vi "PH_Beckhoff_StepMot.evt Call Set Axis Configuration.vi"(0 "i ref in":refnum<vi>, 2 "Instance name":string="N/A", 5 "error in":errorcluster) -> (14 "i ref out":refnum<vi>, 19 "error out":errorcluster)   [LabVIEW 2014, in "PH_Beckhoff_StepMot.lvlib"]
doc: "This VI calls an event by a simple call."
uses:
  PH_Beckhoff_StepMot.lvlib
  instr.lib/Beckhoff/Specials/Step Motor Klemmen/Beckhoff.Step Motor - Motor Configuration.ctl
  instr.lib/Beckhoff/Read and Write Register/Step Motor Klemmen/Beckhoff.Step Motor - Feature Register 1.ctl
  instr.lib/Beckhoff/Read and Write Register/Step Motor Klemmen/Beckhoff.Step Motor - Feature Register 2.ctl
  CS_Core/CSSystem/CoreLib/CoreLib.int 2 byte array.vi
  CS_Core/CSSystem/CoreLib/CoreLib.double 2 byte array.vi
  CS_Core/BaseProcess/BaseProcess.lvlib
  CS_Core/CSSystem/CoreLib/CoreLib.lvlib
  instr.lib/Beckhoff/Beckhoff - Driver np.lvlib
panel:
  in  "Axis":i32=-1
  in  "Step Motor Configuration":T1
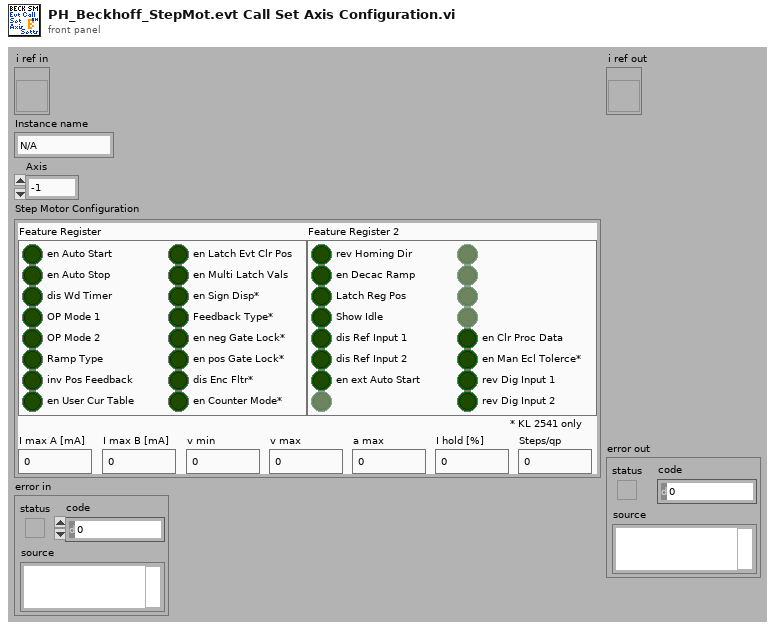
[diagram p1: front panel]
types:
  T1 = typedef "Beckhoff - Driver np.lvlib/Beckhoff.Step Motor - Motor Configuration.ctl" = cluster{"Feature Register":T2, "I max A [mA]":dbl, "I max B [mA]":dbl, "v min":u32, "v max":u32, "a max":u32, "I hold [%]":u32, "Steps/qp":u32, "Feature Register 2":T3}
  T2 = typedef "Beckhoff - Driver np.lvlib/Beckhoff.Step Motor - Feature Register 1.ctl" = cluster{"en Auto Start":bool, "en Auto Stop":bool, "dis Wd Timer":bool, "OP Mode 1":bool, "OP Mode 2":bool, "Ramp Type":bool, "inv Pos Feedback":bool, "en User Cur Table":bool, "en Latch Evt Clr Pos":bool, "en Multi Latch Vals":bool, "en Sign Disp*":bool, "Feedback Type*":bool, "en neg Gate Lock*":bool, "en pos Gate Lock*":bool, "dis Enc Fltr*":bool, "en Counter Mode*":bool}
  T3 = typedef "Beckhoff - Driver np.lvlib/Beckhoff.Step Motor - Feature Register 2.ctl" = cluster{"rev Homing Dir":bool, "en Decac Ramp":bool, "Latch Reg Pos":bool, "Show Idle":bool, "dis Ref Input 1":bool, "dis Ref Input 2":bool, "en ext Auto Start":bool, "N/A":bool, "N/A":bool, "N/A":bool, "N/A":bool, "N/A":bool, "en Clr Proc Data":bool, "en Man Ecl Tolerce*":bool, "rev Dig Input 1":bool, "rev Dig Input 2":bool}
  T4 = typedef "CoreDefs.rawDataType.ctl" = i8[]
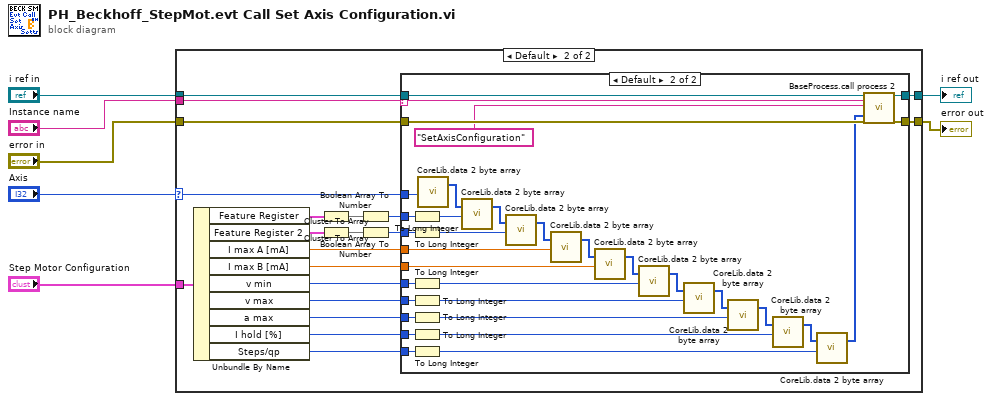
[diagram p0: block diagram]
diagram:
  n1 = case shown="Default" "Axis" {
    selector: "Axis" -> [_ w10]
    tunnel: [w8 w29] -> w7
    tunnel: "error in" -> [w8 w28]
    tunnel: [w9 w27] -> w5
    tunnel: "i ref in" -> [w9 w26]
    tunnel: "Instance name" -> [_ w25]
    tunnel: "Step Motor Configuration" -> [_ w24]
    frame -1 {
    }
    frame Default {
      n2 = Unbundle By Name(w24) -> ("Feature Register"=w23:T2, "Feature Register 2"=w22:T3, "I max A [mA]"=w17:dbl, "I max B [mA]"=w16:dbl, "v min"=w15:u32, "v max"=w14:u32, "a max"=w13:u32, "I hold [%]"=w12:u32, "Steps/qp"=w11:u32)
      n3 = Cluster To Array(cluster=w23) -> (array=w21:bool[])
      n4 = Cluster To Array(cluster=w22) -> (array=w20:bool[])
      n5 = Boolean Array To Number(Boolean array=w21) -> (number=w19:u32)
      n6 = Boolean Array To Number(Boolean array=w20) -> (number=w18:u32)
      n7 = case shown="Default" w25 {
        selector: w25 -> [_ w60]
        tunnel: [w30 w62] -> w29
        tunnel: w28 -> [w30 w61]
        tunnel: [w31 w63] -> w27
        tunnel: w26 -> [w31 w64]
        tunnel: w19 -> [_ w58]
        tunnel: w18 -> [_ w56]
        tunnel: w17 -> [_ w52]
        tunnel: w10 -> [_ w50]
        tunnel: w16 -> [_ w49]
        tunnel: w15 -> [_ w47]
        tunnel: w14 -> [_ w43]
        tunnel: w13 -> [_ w42]
        tunnel: w12 -> [_ w39]
        tunnel: w11 -> [_ w37]
        frame "", "N/A" {
        }
        frame Default {
          n8 = To Long Integer(number=w58) -> (32bit integer=w57:i32)
          n9 = To Long Integer(number=w56) -> (32bit integer=w54:i32)
          n10 = To Long Integer(number=w47) -> (32bit integer=w34:i32)
          n11 = To Long Integer(number=w43) -> (32bit integer=w33:i32)
          n12 = To Long Integer(number=w42) -> (32bit integer=w32:i32)
          n13 = To Long Integer(number=w39) -> (32bit integer=w38:i32)
          n14 = To Long Integer(number=w37) -> (32bit integer=w36:i32)
          n15 = call-poly "CoreLib.data 2 byte array.vi"("i32"=w50) -> ("byteArray out"=w51:T4)  [unwired: 18 in]
          n16 = call-poly "CoreLib.data 2 byte array.vi"("byteArray"=w51, "i32"=w57) -> ("byteArray out"=w55:T4)  [unwired: 17 in]
          n17 = call-poly "CoreLib.data 2 byte array.vi"("byteArray"=w55, "i32"=w54) -> ("byteArray out"=w53:T4)  [unwired: 17 in]
          n18 = call-poly "CoreLib.data 2 byte array.vi"("byteArray"=w53, "f64"=w52) -> ("byteArray out"=w48:T4)  [unwired: 17 in]
          n19 = call-poly "CoreLib.data 2 byte array.vi"("byteArray"=w48, "f64"=w49) -> ("byteArray out"=w46:T4)  [unwired: 17 in]
          n20 = call-poly "CoreLib.data 2 byte array.vi"("byteArray"=w46, "i32"=w34) -> ("byteArray out"=w44:T4)  [unwired: 17 in]
          n21 = call-poly "CoreLib.data 2 byte array.vi"("byteArray"=w44, "i32"=w33) -> ("byteArray out"=w45:T4)  [unwired: 17 in]
          n22 = call-poly "CoreLib.data 2 byte array.vi"("byteArray"=w45, "i32"=w32) -> ("byteArray out"=w40:T4)  [unwired: 17 in]
          n23 = call-poly "CoreLib.data 2 byte array.vi"("byteArray"=w40, "i32"=w38) -> ("byteArray out"=w41:T4)  [unwired: 17 in]
          n24 = call-poly "CoreLib.data 2 byte array.vi"("byteArray"=w41, "i32"=w36) -> ("byteArray out"=w35:T4)  [unwired: 17 in]
          n25 = call "BaseProcess.call process 2.vi"("i ref in"=w64, "Object"=w60, "Selector"="SetAxisConfiguration", "Data"=w35, "error in (no error)"=w61) -> ("i ref out"=w63:refnum<vi>, "error out"=w62:errorcluster)  [unwired: 13 in]
        }
      }
    }
  }
  "error out" <- w7
  "i ref out" <- w5
